vi "Yield.vi"(0 "WAMP Client in":refnum<class "WAMP Client.lvclass">, 5 "Invocation Request ID":u32, 7 "Arguments":variant[](array[variant]), 9 "ArgumentsKw":string, 11 "error in (no error)":errorcluster, 12 "Options":string) -> (4 "WAMP Client out":refnum<class "WAMP Client.lvclass">, 15 "error out":errorcluster)   [LabVIEW 2020, in "WAMP Client.lvclass"]
uses:
  <userlib>/lvwamp/WAMP Client/WAMP Client.lvclass
  <userlib>/lvwamp/WAMP Client/TypeDef/YIELD request data.ctl
  <userlib>/lvwamp/WAMP Client/TypeDef/Internal Message Type.ctl
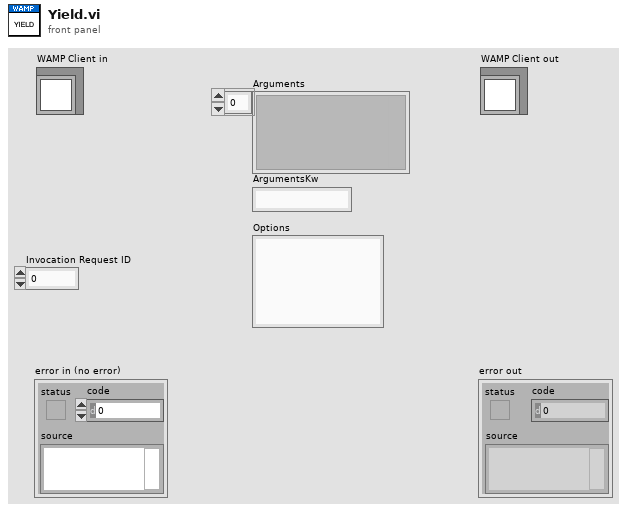
[diagram p1: front panel]
types:
  T1 = typedef "WAMP Client.lvclass/YIELD request data.ctl" = cluster{"Invocation Request ID":u32, "Arguments":variant[], "ArgumentsKw":string, "Options":string}
  T2 = typedef "WAMP Client.lvclass/Internal Message Type.ctl" = enum16{"Subscribe", "Handle Subscribed", "Handle Event", "Unsubscribe", "Handle Unsubscribed", "Publish", "Handled Published", "Goodbye", "Handle Goodbye", "Call", "Handle Result", "Register", "Handle Registered", "Unregister", "Handle Unregistered", "Handle Invocation", "Yield"}
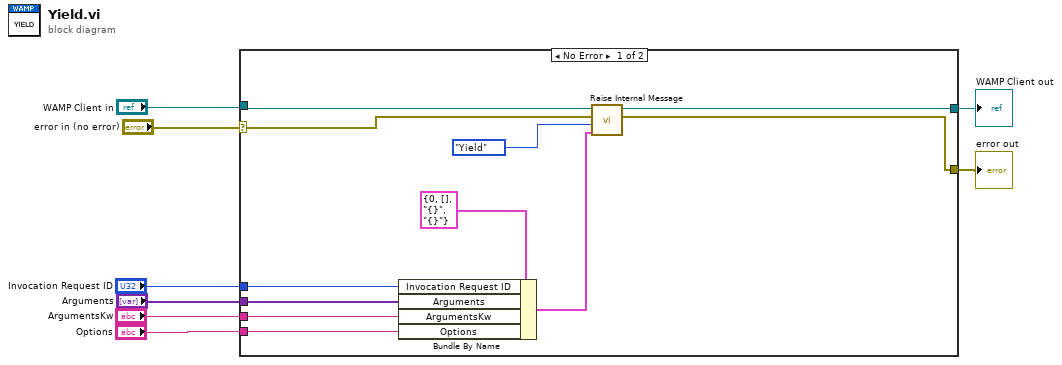
[diagram p0: block diagram]
diagram:
  n1 = case shown="No Error" "error in (no error)" {
    selector: "error in (no error)" -> [w15 w21]
    tunnel: [w16 w21] -> w7
    tunnel: [w18 w20] -> w5
    tunnel: "WAMP Client in" -> [w19 w20]
    tunnel: "ArgumentsKw" -> [w10 _]
    tunnel: "Invocation Request ID" -> [w12 _]
    tunnel: "Arguments" -> [w11 _]
    tunnel: "Options" -> [w9 _]
    frame No Error {
      n2 = Bundle By Name(cluster=T1 {"Invocation Request ID"=0, "Arguments"=[], "ArgumentsKw"="{}", "Options"="{}"} ("Yield request"), "Invocation Request ID"=w12, "Arguments"=w11, "ArgumentsKw"=w10, "Options"=w9) -> (w13:T1)
      n3 = call-dynamic "Raise Internal Message.vi"("Variant"=w13, "Internal Message Type"=Internal_Message_Type."Yield", "error in (no error)"=w15, "WAMP Client in"=w19) -> ("error out"=w16:errorcluster, "WAMP Client out"=w18:refnum<class "WAMP Client.lvclass">)  [unwired: 6 in]
    }
    frame Error {
    }
  }
  "error out" <- w7
  "WAMP Client out" <- w5
